vi "simx Get Object Velocity.vi"(6 "operationMode":i32, 7 "angularVelocity":sgl, 8 "error in (no error)":errorcluster, 9 "linearVelocity":sgl, 10 "objectHandle":i32, 11 "clientID":i32) -> (0 "error out":errorcluster, 1 "linearVelocity out":sgl, 3 "function return":i32, 5 "angularVelocity out":sgl)   [LabVIEW 2019, in "PXL_V-REP.lvlib"]
doc: "EXTAPI_DLLEXPORT simxInt simxGetObjectVelocity(simxInt clientID,simxInt objectHandle,simxFloat* linearVelocity,simxFloat* angularVelocity,simxInt operationMode);"
uses:
  PXL_V-REP.lvlib
  <userlib>/V-REP/remoteApi.dll
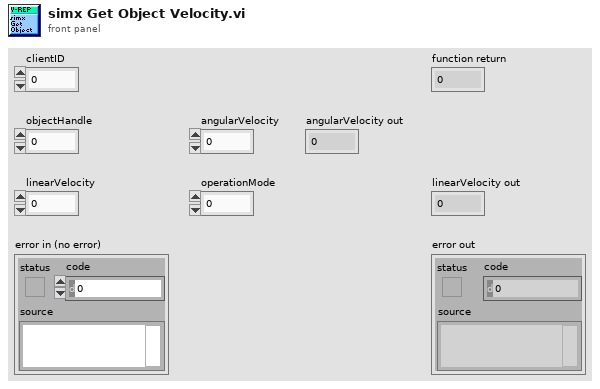
[diagram p1: front panel]
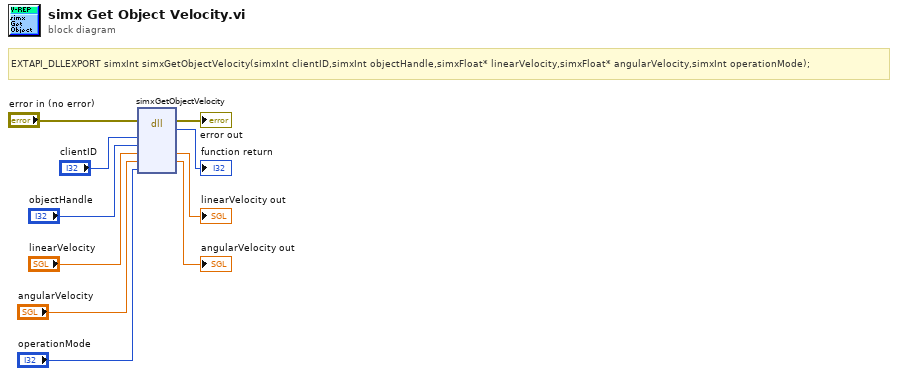
[diagram p0: block diagram]
diagram:
  # "EXTAPI_DLLEXPORT simxInt simxGetObjectVelocity(simxInt clientID,simxInt objectHandle,simxFloat* linearVelocity,simxFloat* angularVelocity,simxInt operationMode);"
  n1 = dll-call lib="C:/Program Files (x86)/National Instruments/LabVIEW 2019/user.lib/V-REP/remoteApi.*" fn="simxGetObjectVelocity"(error in="error in (no error)", "clientID"="clientID", "objectHandle"="objectHandle", "linearVelocity"="linearVelocity", "angularVelocity"="angularVelocity", "operationMode"="operationMode") -> (error out=→"error out":errorcluster, →"function return":i32, "linearVelocity"=→"linearVelocity out":sgl, "angularVelocity"=→"angularVelocity out":sgl)  [unwired: 5 in, 1 out]
